vi "Inspect TBM.vi"(7 "Console Log in":refnum<class "Console Log.lvclass">, 8 "error in":errorcluster, 10 "Module Data In":T1={"TBM-TBM"={"Fiducial Image"={"Image Position"=refnum, "Image Reference"=refnum, "Field of View"={"x(mm)"=0.0, "y(mm)"=0.0}}, "Fiducials"=[]}, "TBM-HDI"={"Fiducial Image"={"Image Position"=refnum, "Image Reference"=refnum, "Field of View"={"x(mm)"=0.0, "y(mm)"=0.0}}, "Fiducials"=[]}, "Address Pads"={"Fiducial Image"={"Image Position"=refnum, "Image Reference"=refnum, "Field of View"={"x(mm)"=0.0, "y(mm)"=0.0}}, "Fiducials"=[]}, "HDI Bond Pad References"=[], "BBM Bond Pad References"=[], "HV-HDI"={"Fiducial Image"={"Image Position"=refnum, "Image Reference"=refnum, "Field of View"={"x(mm)"=0.0, "y(mm)"=0.0}}, "Selected Fiducial"={"Fiducial Image Coordinate"=refnum, "Fiducial Source"=enum."Pattern Recognition"}, "fiducial name"=""}, "HV-BBM"={"Fiducial Image"={"Image Position"=refnum, "Image Reference"=refnum, "Field of View"={"x(mm)"=0.0, "y(mm)"=0.0}}, "Selected Fiducial"={"Fiducial Image Coordinate"=refnum, "Fiducial Source"=enum."Pattern Recognition"}, "fiducial name"=""}, "Chuck"=0, "Slot"=0, "Potting Selection"={"HDI Bond Pads"=[TRUE, TRUE, TRUE, TRUE, TRUE, TRUE, TRUE, TRUE, TRUE, TRUE, TRUE, TRUE, TRUE, TRUE, TRUE, TRUE], "BBM Bond Pads"=[TRUE, TRUE, TRUE, TRUE, TRUE, TRUE, TRUE, TRUE, TRUE, TRUE, TRUE, TRUE, TRUE, TRUE, TRUE, TRUE], "TBM Inner"={"Top"=TRUE, "Left"=TRUE, "Bottom"=TRUE, "Right"=TRUE}, "TBM Outer"={"Top"=TRUE, "Left"=TRUE, "Bottom"=TRUE, "Right"=TRUE}, "Address Pads"={"Top"=TRUE, "Bottom"=TRUE}, "High Voltage"={"HDI"=TRUE, "Sensor"=TRUE}}}, 11 "Potting Procedure in":refnum<class "Potting Procedure.lvclass">) -> (0 "error out":errorcluster, 2 "Module Data Out":T1={"TBM-TBM"={"Fiducial Image"={"Image Position"=refnum, "Image Reference"=refnum, "Field of View"={"x(mm)"=0.0, "y(mm)"=0.0}}, "Fiducials"=[]}, "TBM-HDI"={"Fiducial Image"={"Image Position"=refnum, "Image Reference"=refnum, "Field of View"={"x(mm)"=0.0, "y(mm)"=0.0}}, "Fiducials"=[]}, "Address Pads"={"Fiducial Image"={"Image Position"=refnum, "Image Reference"=refnum, "Field of View"={"x(mm)"=0.0, "y(mm)"=0.0}}, "Fiducials"=[]}, "HDI Bond Pad References"=[], "BBM Bond Pad References"=[], "HV-HDI"={"Fiducial Image"={"Image Position"=refnum, "Image Reference"=refnum, "Field of View"={"x(mm)"=0.0, "y(mm)"=0.0}}, "Selected Fiducial"={"Fiducial Image Coordinate"=refnum, "Fiducial Source"=enum."Pattern Recognition"}, "fiducial name"=""}, "HV-BBM"={"Fiducial Image"={"Image Position"=refnum, "Image Reference"=refnum, "Field of View"={"x(mm)"=0.0, "y(mm)"=0.0}}, "Selected Fiducial"={"Fiducial Image Coordinate"=refnum, "Fiducial Source"=enum."Pattern Recognition"}, "fiducial name"=""}, "Chuck"=0, "Slot"=0, "Potting Selection"={"HDI Bond Pads"=[TRUE, TRUE, TRUE, TRUE, TRUE, TRUE, TRUE, TRUE, TRUE, TRUE, TRUE, TRUE, TRUE, TRUE, TRUE, TRUE], "BBM Bond Pads"=[TRUE, TRUE, TRUE, TRUE, TRUE, TRUE, TRUE, TRUE, TRUE, TRUE, TRUE, TRUE, TRUE, TRUE, TRUE, TRUE], "TBM Inner"={"Top"=TRUE, "Left"=TRUE, "Bottom"=TRUE, "Right"=TRUE}, "TBM Outer"={"Top"=TRUE, "Left"=TRUE, "Bottom"=TRUE, "Right"=TRUE}, "Address Pads"={"Top"=TRUE, "Bottom"=TRUE}, "High Voltage"={"HDI"=TRUE, "Sensor"=TRUE}}}, 3 "Potting Procedure out":refnum<class "Potting Procedure.lvclass">, 5 "Console Log out":refnum<class "Console Log.lvclass">)   [LabVIEW 2011, in "Potting Procedure.lvclass"]
uses:
  Potting Procedure.lvclass
  UI Classes/Console Log/Console Log.lvclass
  Type Definitions/Inspect Modules - Module.ctl
  Shared Components/Vec3d Class/Vec3d Class.lvclass
  Shared Components/Utils/Type Definitions/Multi-Fiducial Image.ctl
  Shared Components/Utils/Type Definitions/Physical Image.ctl
  <vilib>/vision/Image Controls.llb/IMAQ Image.ctl
  Shared Components/Utils/Type Definitions/Fiducial with Source.ctl
  Shared Components/Utils/Type Definitions/Fiducial Image.ctl
  Shared Components/Gantry Class/Gantry Class.lvclass
  Shared Components/WorkTable Class/WorkTable Class.lvclass
  Shared Components/CameraTool Class/Take Outline Image.vi
  Shared Components/CameraTool Class/CameraTool Class.lvclass
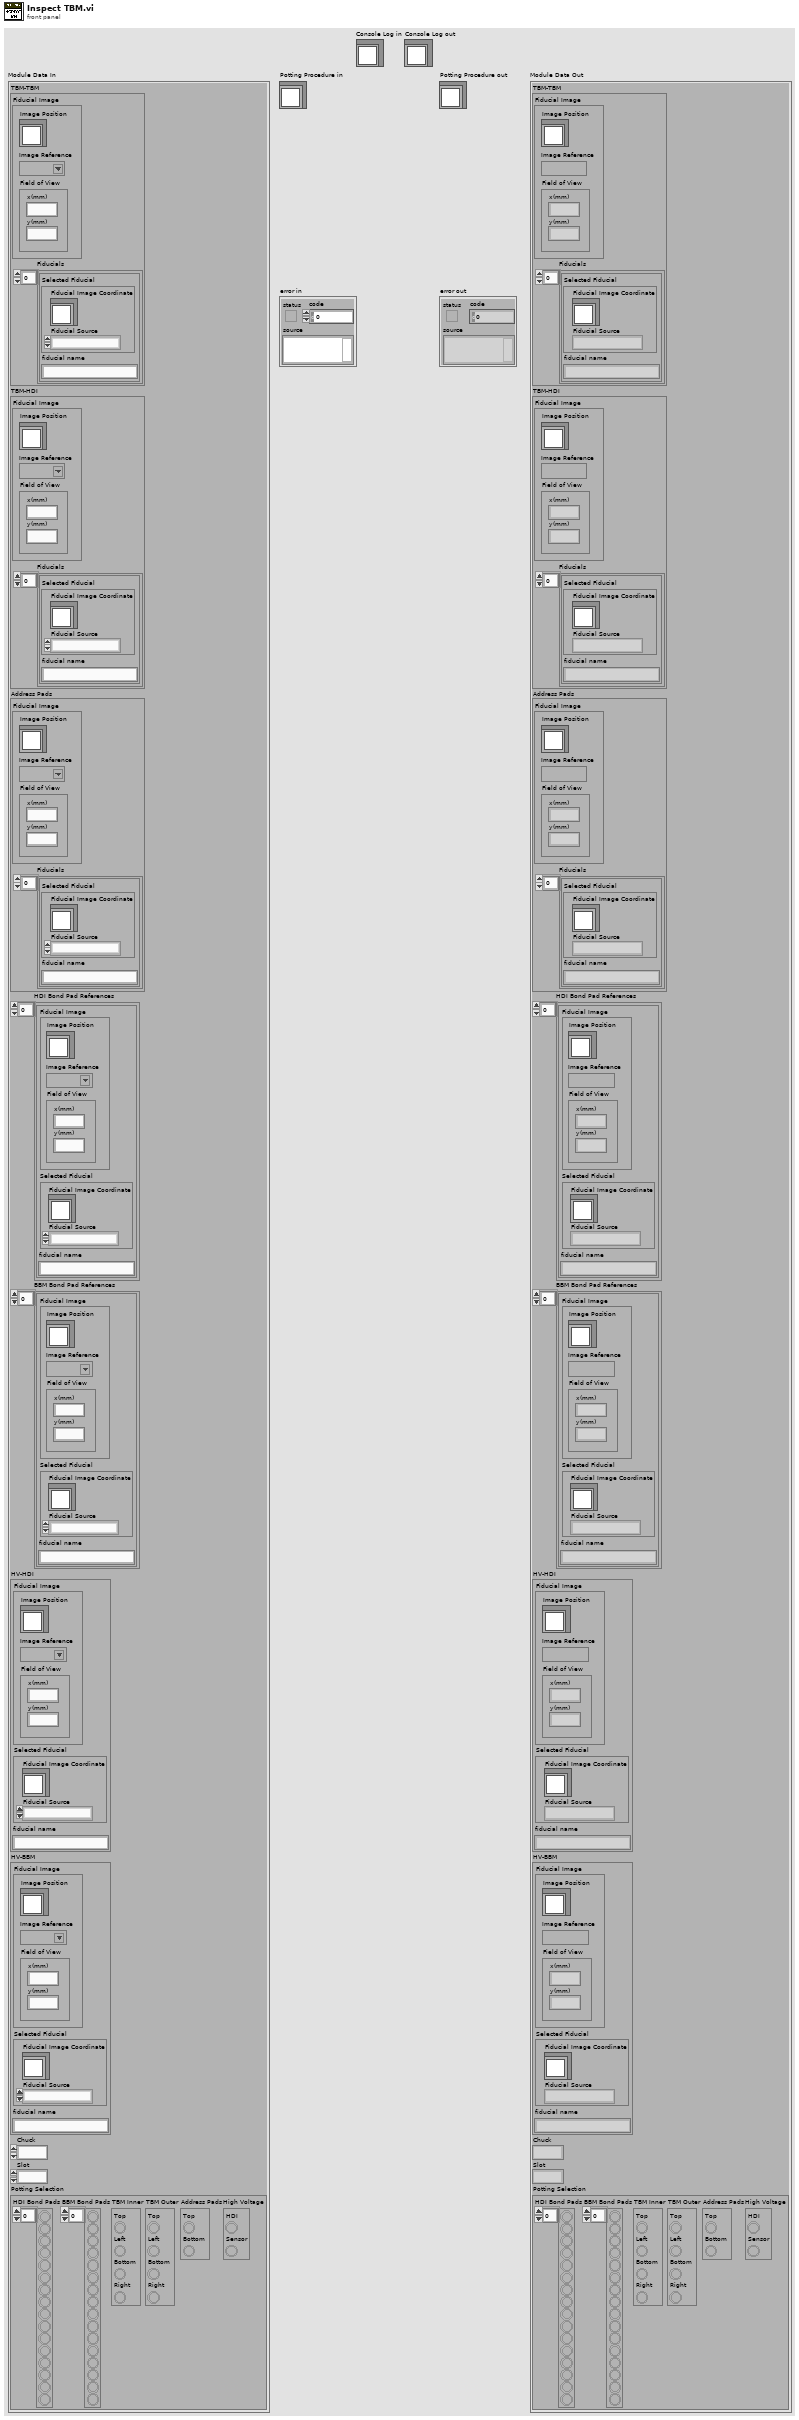
[diagram p1: front panel]
types:
  T1 = typedef "Inspect Modules - Module.ctl" = cluster{"TBM-TBM":T2, "TBM-HDI":T2, "Address Pads":T2, "HDI Bond Pad References":T6[], "BBM Bond Pad References":T6[], "HV-HDI":T6, "HV-BBM":T6, "Chuck":i32, "Slot":i32, "Potting Selection":cluster{"HDI Bond Pads":bool[], "BBM Bond Pads":bool[], "TBM Inner":cluster{"Top":bool, "Left":bool, "Bottom":bool, "Right":bool}, "TBM Outer":cluster{"Top":bool, "Left":bool, "Bottom":bool, "Right":bool}, "Address Pads":cluster{"Top":bool, "Bottom":bool}, "High Voltage":cluster{"HDI":bool, "Sensor":bool}}}
  T2 = typedef "Multi-Fiducial Image.ctl" = cluster{"Fiducial Image":T3, "Fiducials":cluster{"Selected Fiducial":T5, "fiducial name":string}[]}
  T3 = typedef "Physical Image.ctl" = cluster{"Image Position":refnum<class "Vec3d Class.lvclass">, "Image Reference":T4, "Field of View":cluster{"x(mm)":dbl, "y(mm)":dbl}}
  T4 = typedef "IMAQ Image.ctl" = refnum<image>
  T5 = typedef "Fiducial with Source.ctl" = cluster{"Fiducial Image Coordinate":refnum<class "Vec3d Class.lvclass">, "Fiducial Source":enum16{"Pattern Recognition", "User", "Error", "Default"}}
  T6 = typedef "Fiducial Image.ctl" = cluster{"Fiducial Image":T3, "Selected Fiducial":T5, "fiducial name":string}
  T7 = enum16{"Pattern Recognition", "User", "Error", "Default"}
  T8 = cluster{"Selected Fiducial":T5, "fiducial name":string}
  T9 = typedef "Worktable_Module Slot.ctl" = cluster{"Slot State":enum16{"Empty", "Unglued", "Stamped", "PartOnTop", "Weighted", "Unpotted", "Potted"}, "BBM Type":enum16{"None", "BBM", "GlassSlide"}, "HDI Type":enum16{"None", "HDI", "Polyimide"}, "Vacuum Channel":u8, "Location/Orientation BBM":T10, "Location/Orientation HDI":T10, "S/N":string}
  T10 = typedef "Position_Orientation.ctl" = cluster{"Center":refnum<class "Vec3d Class.lvclass">, "Orientation":refnum<class "Orient3d Class.lvclass">}
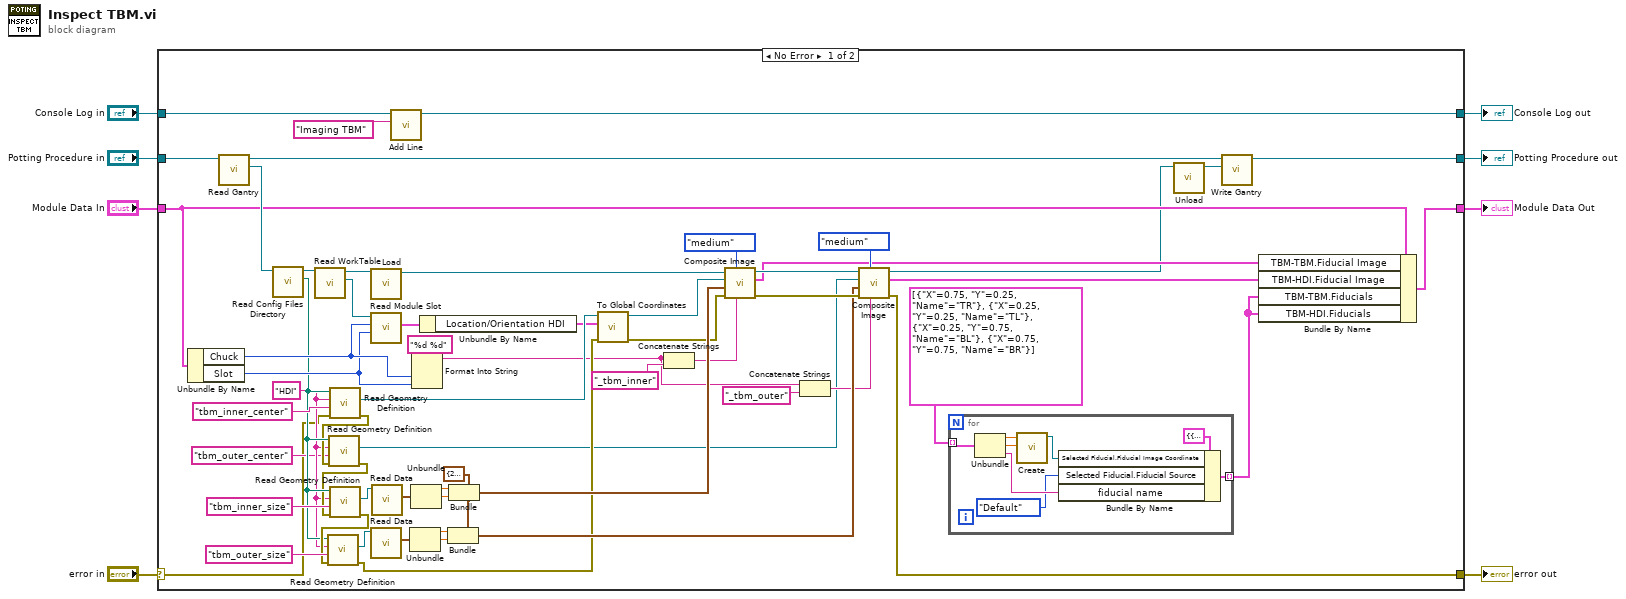
[diagram p0: block diagram]
diagram:
  n1 = case shown="No Error" "error in" {
    selector: "error in" -> [w9 w80]
    tunnel: [w37 w80] -> w7
    tunnel: [w21 w79] -> w5
    tunnel: "Potting Procedure in" -> [w68 w79]
    tunnel: "Module Data In" -> [w28 w78]
    tunnel: [w23 w78] -> w1
    tunnel: "Console Log in" -> [w18 w77]
    tunnel: [w17 w77] -> w3
    frame No Error {
      w48 = cluster{"Size-X(mm)":dbl, "Size-Y(mm)":dbl} {"Size-X(mm)"=20.0, "Size-Y(mm)"=20.0} ("Field of View")
      w12 = "HDI" ("Part")
      n2 = Unbundle By Name(w28) -> ("Chuck"=w30:i32, "Slot"=w29:i32)
      n3 = call-dynamic "Read Gantry.vi"("Potting Procedure in"=w68) -> ("Gantry"=w65:refnum<class "Gantry Class.lvclass">, "Potting Procedure out"=w20:refnum<class "Potting Procedure.lvclass">)  [unwired: 8 in, 1 out]
      n4 = call-dynamic "Read Config Files Directory.vi"("Gantry Class in"=w65) -> ("Config Files Directory"=w15:path, "Gantry Class out"=w46:refnum<class "Gantry Class.lvclass">)  [unwired: 8 in, 1 out]
      n5 = call-dynamic "Read WorkTable.vi"("Gantry Class in"=w46) -> ("WorkTable Class.lvclass"=w44:refnum<class "WorkTable Class.lvclass">, "Gantry Class out"=w45:refnum<class "Gantry Class.lvclass">)  [unwired: 8 in, 1 out]
      n6 = call "Read Geometry Definition.vi"("error in"=w9, "Feature"="tbm_inner_center", "Part"=w12, "Config Location"=w15) -> ("error out"=w13:errorcluster, "Feature Coordinates"=w42:refnum<class "Vec3d Class.lvclass">)  [unwired: 6 in]
      n7 = call "Read Geometry Definition.vi"("error in"=w13, "Feature"="tbm_outer_center", "Part"=w12, "Config Location"=w15) -> ("error out"=w14:errorcluster, "Feature Coordinates"=w10:refnum<class "Vec3d Class.lvclass">)  [unwired: 6 in]
      n8 = call "Read Geometry Definition.vi"("error in"=w14, "Feature"="tbm_inner_size", "Part"=w12, "Config Location"=w15) -> ("error out"=w61:errorcluster, "Feature Coordinates"=w57:refnum<class "Vec3d Class.lvclass">)  [unwired: 6 in]
      n9 = call "Read Geometry Definition.vi"("error in"=w61, "Feature"="tbm_outer_size", "Part"=w12, "Config Location"=w15) -> ("error out"=w40:errorcluster, "Feature Coordinates"=w49:refnum<class "Vec3d Class.lvclass">)  [unwired: 6 in]
      n10 = call "Load.vi"("Gantry In"=w45) -> ("CameraTool out"=w67:refnum<class "CameraTool Class.lvclass">)  [unwired: 9 in, 1 out]
      n11 = call-dynamic "Read Module Slot.vi"("slot"=w29, "chuck"=w30, "WorkTable in"=w44) -> ("Module Slot"=w43:T9)  [unwired: 6 in, 2 out]
      n12 = call-dynamic "Read Data.vi"("Vec3d Class in"=w49) -> ("Data"=w52:cluster{"X":dbl, "Y":dbl, "Z":dbl})  [unwired: 8 in, 2 out]
      n13 = call-dynamic "Read Data.vi"("Vec3d Class in"=w57) -> ("Data"=w56:cluster{"X":dbl, "Y":dbl, "Z":dbl})  [unwired: 8 in, 2 out]
      n14 = call "Add Line.vi"("String"="Imaging TBM", "Console Log in"=w18) -> ("Console Log out"=w17:refnum<class "Console Log.lvclass">)  [unwired: 8 in, 1 out]
      n15 = Unbundle(w52) -> ("X"=w51:dbl, "Y"=w50:dbl)  [unwired: 1 out]
      n16 = Unbundle(w56) -> ("X"=w55:dbl, "Y"=w54:dbl)  [unwired: 1 out]
      n17 = Format Into String(format string="%d %d", w30, w29) -> (resulting string=w33:string)  [unwired: 2 in, 1 out]
      n18 = Unbundle By Name(w43) -> ("Location/Orientation HDI"=w41:T10)
      n19 = Bundle(cluster=w48, "Size-X(mm)"=w51, "Size-Y(mm)"=w50) -> (w47:cluster{"Size-X(mm)":dbl, "Size-Y(mm)":dbl})
      n20 = Bundle(cluster=w48, "Size-X(mm)"=w55, "Size-Y(mm)"=w54) -> (w53:cluster{"Size-X(mm)":dbl, "Size-Y(mm)":dbl})
      n21 = call "To Global Coordinates.vi"("error in"=w40, "Center/Orientation"=w41, "Local Coordinates"=w42) -> ("error out"=w39:errorcluster, "Global Coordinates"=w38:refnum<class "Vec3d Class.lvclass">)  [unwired: 7 in]
      n22 = Concatenate Strings(w33, "_tbm_inner" ("string")) -> (w32:string)
      n23 = call-poly "Composite Image.vi"("Image Name"=w32, "Quality"=enum16{"perfect", "medium", "low"}."medium", "error in"=w39, "Field of View"=w53, "Image Center"=w38, "CameraTool in"=w67) -> ("error out"=w58:errorcluster, "Physical Image"=w27:T3, "CameraTool out"=w60:refnum<class "CameraTool Class.lvclass">)  [unwired: 3 in]
      n24 = Concatenate Strings(w33, "_tbm_outer" ("string")) -> (w31:string)
      n25 = call-poly "Composite Image.vi"("Image Name"=w31, "Quality"=enum16{"perfect", "medium", "low"}."medium", "error in"=w58, "Field of View"=w47, "Image Center"=w10, "CameraTool in"=w60) -> ("error out"=w37:errorcluster, "Physical Image"=w26:T3, "CameraTool out"=w22:refnum<class "CameraTool Class.lvclass">)  [unwired: 3 in]
      n26 = for {
        tunnel: cluster{"X":dbl, "Y":dbl, "Name":string}[] [{"X"=0.75, "Y"=0.25, "Name"="TR"}, {"X"=0.25, "Y"=0.25, "Name"="TL"}, {"X"=0.25, "Y"=0.75, "Name"="BL"}, {"X"=0.75, "Y"=0.75, "Name"="BR"}] -> [w75] mode=indexing
        tunnel: [w69] -> w24 mode=indexing
        n27 = Unbundle(w75) -> ("X"=w73:dbl, "Y"=w74:dbl, "Name"=w71:string)
        n28 = call "Create.vi"("Y"=w74, "X"=w73) -> ("Vec3d Class out"=w72:refnum<class "Vec3d Class.lvclass">)  [unwired: 8 in, 1 out]
        n29 = Bundle By Name(cluster=T8 {"Selected Fiducial"={"Fiducial Image Coordinate"=refnum, "Fiducial Source"=enum."Pattern Recognition"}, "fiducial name"=""} ("Fiducial"), "Selected Fiducial.Fiducial Image Coordinate"=w72, "Selected Fiducial.Fiducial Source"=T7."Default", "fiducial name"=w71) -> (w69:T8)
      }
      n30 = call "Unload.vi"("CameraTool in"=w22) -> ("Gantry out"=w19:refnum<class "Gantry Class.lvclass">)  [unwired: 9 in, 1 out]
      n31 = call-dynamic "Write Gantry.vi"("Gantry"=w19, "Potting Procedure in"=w20) -> ("Potting Procedure out"=w21:refnum<class "Potting Procedure.lvclass">)  [unwired: 8 in, 1 out]
      n32 = Bundle By Name(cluster=w28, "TBM-TBM.Fiducial Image"=w27, "TBM-HDI.Fiducial Image"=w26, "TBM-TBM.Fiducials"=w24, "TBM-HDI.Fiducials"=w24) -> (w23:T1)
    }
    frame Error {
    }
  }
  "error out" <- w7
  "Potting Procedure out" <- w5
  "Console Log out" <- w3
  "Module Data Out" <- w1
